vi "关键参数转data(子VI).vi"(10 "改变?":bool, 11 "关键参数":T1) -> (3 "数组":string[][](array[string]))   [LabVIEW 2016, in "数据传输系统.lvlib"]
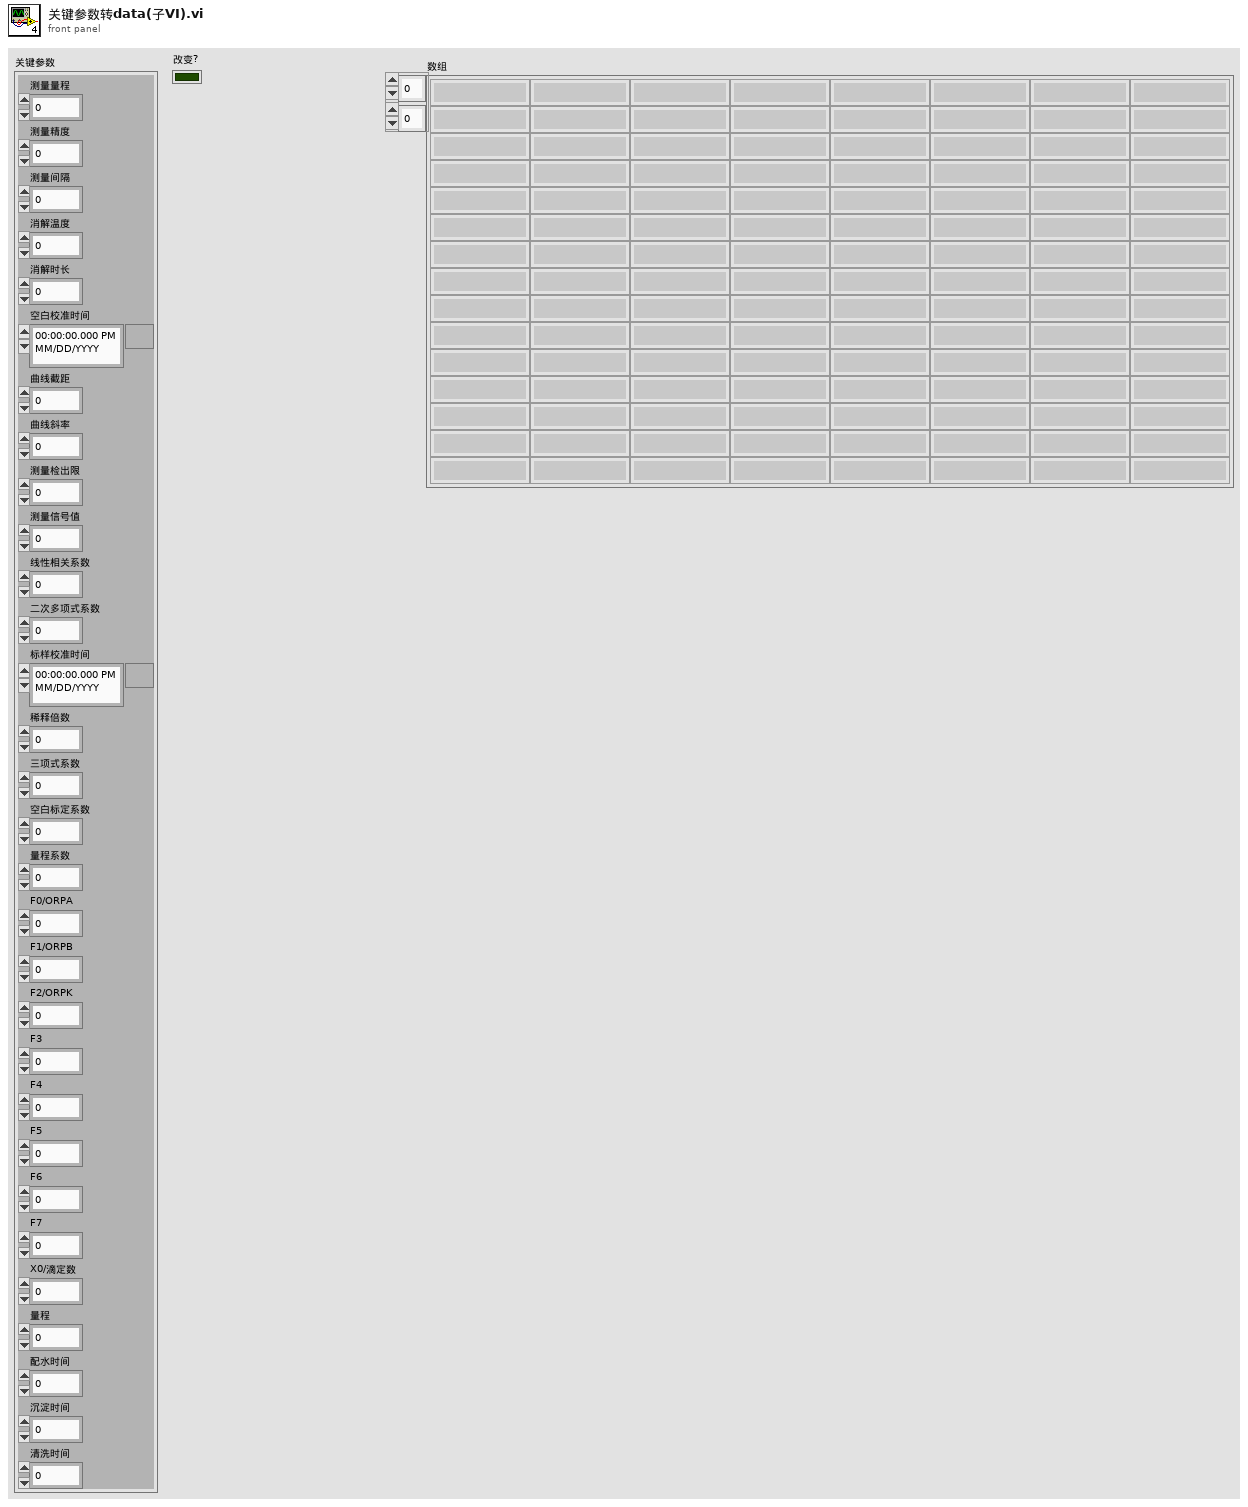
[diagram p1: front panel]
types:
  T1 = cluster{"测量量程":dbl, "测量精度":dbl, "测量间隔":dbl, "消解温度":dbl, "消解时长":dbl, "空白校准时间":timestamp, "曲线截距":dbl, "曲线斜率":dbl, "测量检出限":dbl, "测量信号值":dbl, "线性相关系数":dbl, "二次多项式系数":dbl, "标样校准时间":timestamp, "稀释倍数":dbl, "三项式系数":dbl, "空白标定系数":dbl, "量程系数":dbl, "F0/ORPA":dbl, "F1/ORPB":dbl, "F2/ORPK":dbl, "F3":dbl, "F4":dbl, "F5":dbl, "F6":dbl, "F7":dbl, "X0/滴定数":dbl, "量程":dbl, "配水时间":dbl, "沉淀时间":dbl, "清洗时间":dbl}
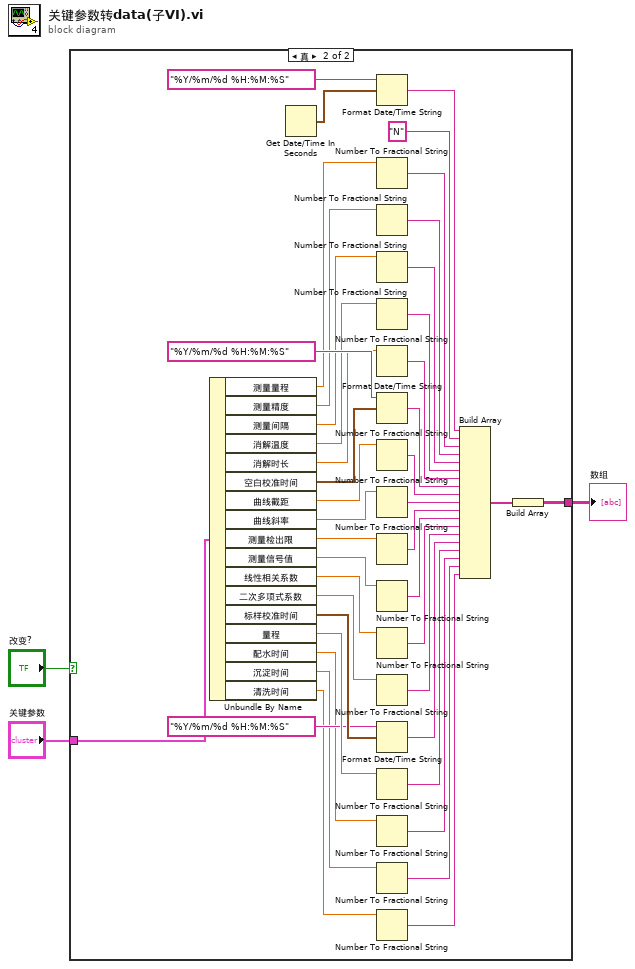
[diagram p0: block diagram]
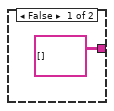
[diagram p2: hidden frame]
diagram:
  n1 = case shown="真" "改变?" {
    tunnel: [string[][] [] w47] -> w3
    tunnel: "关键参数" -> [_ w11]
    frame False {
    }
    frame True {
      n2 = Unbundle By Name(w11) -> ("测量量程"=w12:dbl, "测量精度"=w18:dbl, "测量间隔"=w20:dbl, "消解温度"=w22:dbl, "消解时长"=w24:dbl, "空白校准时间"=w27:timestamp, "曲线截距"=w29:dbl, "曲线斜率"=w30:dbl, "测量检出限"=w31:dbl, "测量信号值"=w32:dbl, "线性相关系数"=w33:dbl, "二次多项式系数"=w34:dbl, "标样校准时间"=w36:timestamp, "量程"=w37:dbl, "配水时间"=w10:dbl, "沉淀时间"=w9:dbl, "清洗时间"=w8:dbl)
      n3 = Get Date/Time In Seconds() -> (seconds since 1Jan1904=w14:timestamp)
      n4 = Format Date/Time String(time format string (%c)="%Y/%m/%d %H:%M:%S" ("时间格式字符串(%c)"), seconds (now)=w14) -> (date/time string=w15:string)  [unwired: 1 in]
      n5 = Number To Fractional String(number=w12) -> (F-format string=w17:string)  [unwired: 3 in]
      n6 = Number To Fractional String(number=w18) -> (F-format string=w19:string)  [unwired: 3 in]
      n7 = Number To Fractional String(number=w20) -> (F-format string=w21:string)  [unwired: 3 in]
      n8 = Number To Fractional String(number=w22) -> (F-format string=w23:string)  [unwired: 3 in]
      n9 = Number To Fractional String(number=w24) -> (F-format string=w25:string)  [unwired: 3 in]
      n10 = Format Date/Time String(time format string (%c)="%Y/%m/%d %H:%M:%S" ("时间格式字符串(%c)"), seconds (now)=w27) -> (date/time string=w28:string)  [unwired: 1 in]
      n11 = Number To Fractional String(number=w29) -> (F-format string=w38:string)  [unwired: 3 in]
      n12 = Number To Fractional String(number=w30) -> (F-format string=w39:string)  [unwired: 3 in]
      n13 = Number To Fractional String(number=w31) -> (F-format string=w40:string)  [unwired: 3 in]
      n14 = Number To Fractional String(number=w32) -> (F-format string=w41:string)  [unwired: 3 in]
      n15 = Number To Fractional String(number=w33) -> (F-format string=w42:string)  [unwired: 3 in]
      n16 = Number To Fractional String(number=w34) -> (F-format string=w43:string)  [unwired: 3 in]
      n17 = Format Date/Time String(time format string (%c)="%Y/%m/%d %H:%M:%S" ("时间格式字符串(%c)"), seconds (now)=w36) -> (date/time string=w44:string)  [unwired: 1 in]
      n18 = Number To Fractional String(number=w37) -> (F-format string=w45:string)  [unwired: 3 in]
      n19 = Number To Fractional String(number=w10) -> (F-format string=w7:string)  [unwired: 3 in]
      n20 = Number To Fractional String(number=w9) -> (F-format string=w6:string)  [unwired: 3 in]
      n21 = Number To Fractional String(number=w8) -> (F-format string=w5:string)  [unwired: 3 in]
      n22 = Build Array(w15, "N", w17, w19, w21, w23, w25, w28, w38, w39, w40, w41, w42, w43, w44, w45, w7, w6, w5) -> (w46:string[])
      n23 = Build Array(w46) -> (w47:string[][])
    }
  }
  "数组" <- w3
